vi "DAC Run.vi"(8 "error in":errorcluster, 11 "DAC Inverter in":refnum<class "DAC Inverter.lvclass">) -> (0 "error out":errorcluster, 3 "DAC Inverter out":refnum<class "DAC Inverter.lvclass">)   [LabVIEW 2019, in "DAC.lvlib" / "DAC Inverter.lvclass"]
uses:
  DAC Inverter.lvclass
  C:/Users/wg/Documents/LV_Projects/test-stand/App/DAC/DAC.lvclass
  DAC.lvclass/DAC.ctl
  Results/Results Method.ctl
  Results/DeepU Results/DeepU Results.lvclass
  DAC Inverter.lvclass/DAC Inverter.ctl
  DAC.lvclass
  Results/Results.lvlib
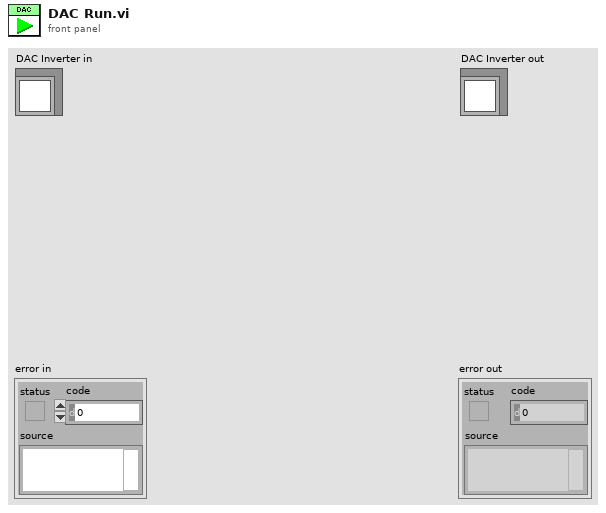
[diagram p1: front panel]
types:
  T1 = typedef "Results.lvlib/Results Method.ctl" = enum16{"Get", "Set"}
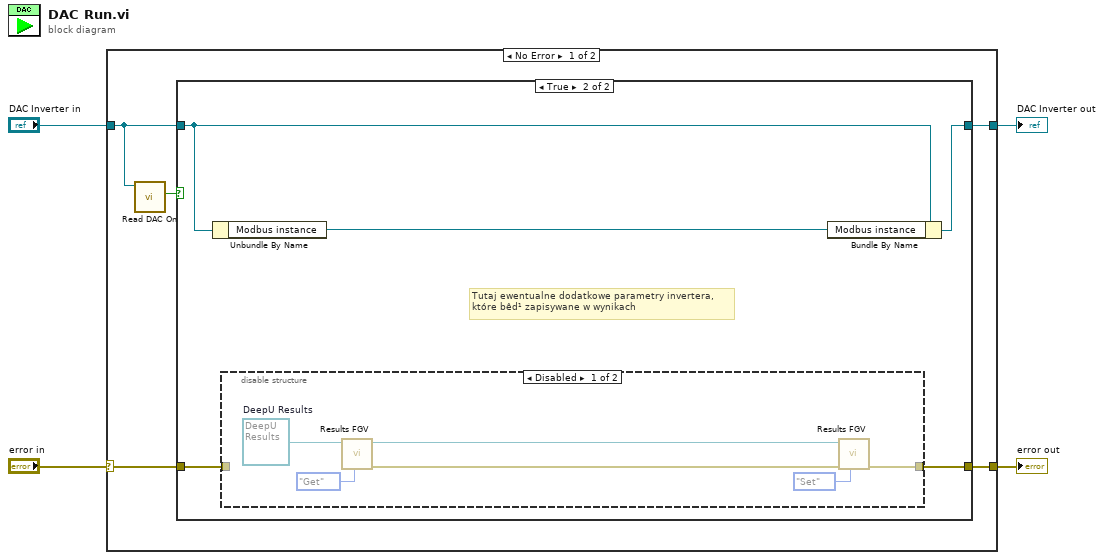
[diagram p0: block diagram]
diagram:
  n1 = case shown="No Error" "error in" {
    selector: "error in" -> [w7 w25]
    tunnel: [w6 w25] -> w2
    tunnel: [w8 w24] -> w1
    tunnel: "DAC Inverter in" -> [w5 w24]
    frame No Error {
      n2 = call "Read DAC On.vi"("DAC in"=w5) -> ("DAC On"=w9:bool)  [unwired: 8 in, 2 out]
      n3 = case shown="True" w9 {
        tunnel: w5 -> [w11 w16]
        tunnel: [w11 w14] -> w8
        tunnel: w7 -> [w10 w12]
        tunnel: [w10 w15] -> w6
        frame False {
        }
        frame True {
          # "Tutaj ewentualne dodatkowe parametry invertera,\nktóre bêd¹ zapisywane w wynikach"
          n4 = Unbundle By Name(w16) -> ("Modbus instance"=w13:refnum<class "Modbus Master.lvclass">)
          n5 = disable-structure shown="Disabled" {
            disable-tunnel: [w19 w23] -> w15
            disable-tunnel: w12 -> [_ w23]
            frame Disabled {
              w22 = refnum<class "DeepU Results.lvclass"> refnum  # DeepU Results
              n6 = call-dynamic "Results FGV.vi"("Method"=Results_Method."Get", "DeepU Results in"=w22) -> ("error out"=w17:errorcluster, "DeepU Results out"=w18:refnum<class "DeepU Results.lvclass">)  [unwired: 8 in]
              n7 = call-dynamic "Results FGV.vi"("Method"=Results_Method."Set", "error in"=w17, "DeepU Results in"=w18) -> ("error out"=w19:errorcluster)  [unwired: 7 in, 1 out]
            }
            frame Enabled {
            }
          }
          n8 = Bundle By Name(cluster=w16, "Modbus instance"=w13) -> (w14:refnum<class "DAC Inverter.lvclass">)
        }
      }
    }
    frame Error {
    }
  }
  "error out" <- w2
  "DAC Inverter out" <- w1
